vi "wfm_createChan.vi"(8 "error in":errorcluster, 10 "Sensitivity":sgl[](array[numeric]), 11 "Dynamic FPGA VI Reference 2":T1) -> (0 "error out":errorcluster, 3 "Dynamic FPGA VI Reference":T1)   [LabVIEW 2015]
uses:
  <vilib>/addons/InsightCM/Devices/Shared/cRIOWfmAcq/subVIs/RIO Wfm Cust Ctrls/rwfm_DynamicFPGAref2.ctl
  <vilib>/Utility/error.llb/Error Cluster From Error Code.vi
  <vilib>/rvi/errors/niLvFpgaAdjustHostInterfaceError.vi
  <vilib>/rvi/interface/nirviReadWriteControl/nirviReadWriteControl.xnode
  <vilib>/addons/InsightCM/Devices/Shared/cRIOWfmAcq/cRIOWfmLib.lvlib
  <vilib>/rvi/interface/Simulation/niFpgaSimulationCallBeginRW.vi
  NiFpgaLv.dll
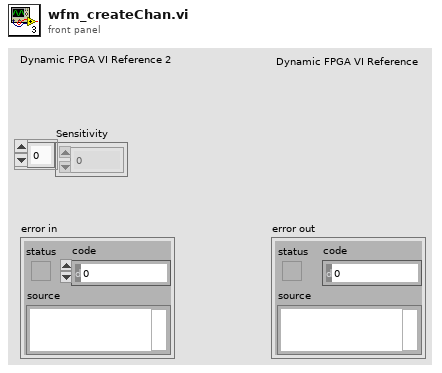
[diagram p1: front panel]
types:
  T1 = typedef "cRIOWfmLib.lvlib/rwfm_DynamicFPGAref2.ctl" = refnum<k20>
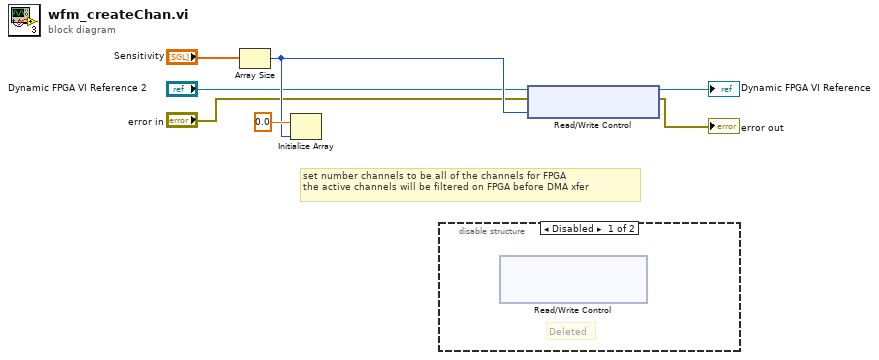
[diagram p0: block diagram]
diagram:
  # "set number channels to be all of the channels for FPGA\nthe active channels will be filtered on FPGA before DMA xfer"
  n1 = Array Size(array="Sensitivity") -> (size(s)=w3:i32)
  n2 = Initialize Array(sgl 0.0, w3) -> ()  [unwired: 1 out]
  n3 = disable-structure shown="Disabled" {
    frame Disabled {
      # "Deleted"
      n4 = xnode "Read/Write Control"() -> ()  [unwired: 4 in, 2 out]
    }
    frame Enabled {
    }
  }
  n5 = xnode "Read/Write Control"("FPGA VI Reference In"="Dynamic FPGA VI Reference 2", "error in"="error in", "Total Avail Channels"=w3) -> ("FPGA VI Reference Out"=→"Dynamic FPGA VI Reference":T1, "error out"=→"error out":errorcluster)
